vi "Test Double Factory.vi"() -> ()   [LabVIEW 2020, in "Test Double Factory.lvclass"]
uses:
  Test Double Factory.lvclass
panel:
  out "Test Double Factory out":refnum<class "Test Double Factory.lvclass">
  in  "Test Double Factory.lvclass":refnum<class "Test Double Factory.lvclass">
  out "error out":errorcluster
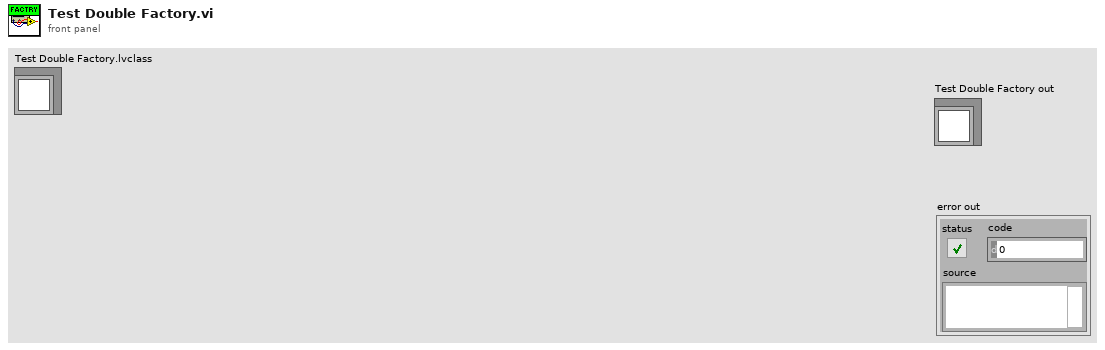
[diagram p1: front panel]
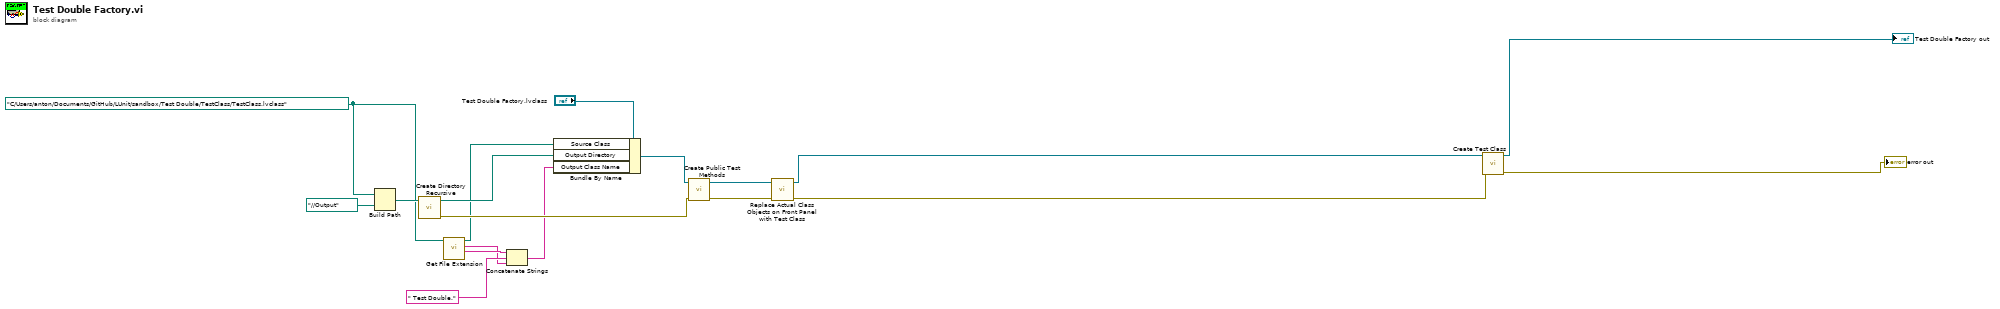
[diagram p0: block diagram]
diagram:
  w4 = path "C:/Users/anton/Documents/GitHub/LUnit/sandbox/Test Double/TestClass/TestClass.lvclass" ("name or relative path")
  n1 = Build Path(base path=w4, name or relative path=path "../../Output") -> (appended path=w15:path)
  n2 = call <vilib>:"Create Directory Recursive.vi"("directory"=w15) -> ("error out"=w9:errorcluster, "directory copy"=w13:path)  [unwired: 4 in, 1 out]
  n3 = call <vilib>:"Get File Extension.vi"("file"=w4) -> ("filename without extension"=w18:string, "lowercase file extension"=w16:string, "dup file"=w3:path)  [unwired: 6 in, 2 out]
  n4 = Concatenate Strings(w18, " Test Double." ("string"), w16) -> (w2:string)
  n5 = Bundle By Name(cluster="Test Double Factory.lvclass", "Source Class"=w3, "Output Directory"=w13, "Output Class Name"=w2) -> (w11:refnum<class "Test Double Factory.lvclass">)
  n6 = call "Create Public Test Methods.vi"("error in (no error)"=w9, "Test Double Factory in"=w11) -> ("error out"=w8:errorcluster, "Test Double Factory out"=w6:refnum<class "Test Double Factory.lvclass">)  [unwired: 8 in]
  n7 = call "Replace Actual Class Objects on Front Panel with Test Class.vi"("error in (no error)"=w8, "Test Double Factory in"=w6) -> ("error out"=w7:errorcluster, "Test Double Factory out"=w5:refnum<class "Test Double Factory.lvclass">)  [unwired: 8 in]
  n8 = call "Create Test Class.vi"("error in (no error)"=w7, "Test Double Factory in"=w5) -> ("error out"=→"error out":errorcluster, "Test Double Factory out"=→"Test Double Factory out":refnum<class "Test Double Factory.lvclass">)  [unwired: 8 in]
